vi "myRIO_BRig_Host_formatData_getPaths_label.vi"(11 "input_filePath":string) -> (2 "output_filePath_label":string)   [LabVIEW 2014]
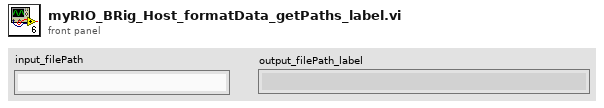
[diagram p1: front panel]
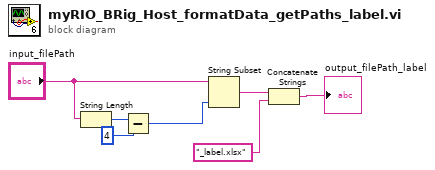
[diagram p0: block diagram]
diagram:
  n1 = String Length(string="input_filePath") -> (length=w7:i32)
  n2 = Subtract(x=w7, y=4) -> (x-y=w4:i32)
  n3 = String Subset(string="input_filePath", length (rest)=w4) -> (substring=w3:string)  [unwired: 1 in]
  n4 = Concatenate Strings(w3, "_label.xlsx" ("string")) -> (→"output_filePath_label":string)
